vi "acquire multi waves init subvi.vi"(10 "Enum in":enum16{"Idle", "Start"}(ring), 11 "VISA Refnum in":refnum<visa-resource-name>) -> (0 "error out":errorcluster, 1 "read buffer":string, 2 "Enum out":enum16{"Idle", "Start"}(ring), 3 "VISA Refnum out":refnum<visa-resource-name>)   [LabVIEW 2013]
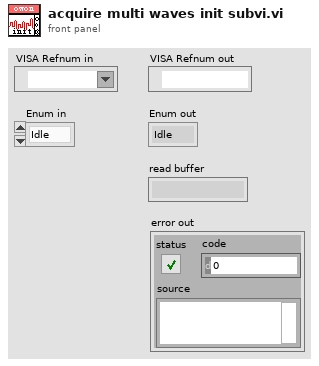
[diagram p1: front panel]
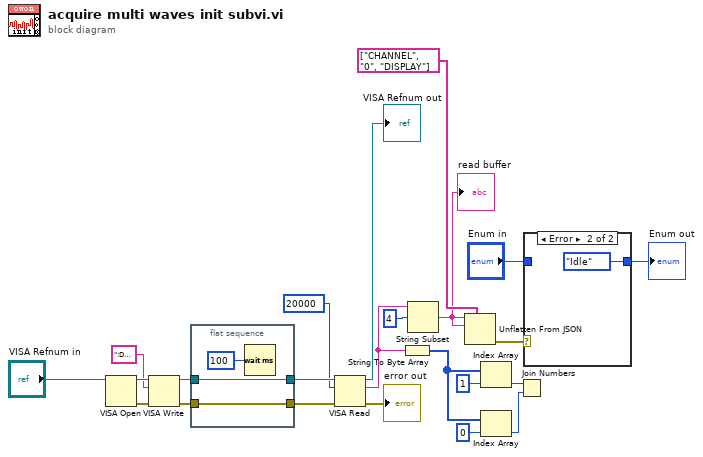
[diagram p0: block diagram]
diagram:
  n1 = VISA Open(VISA resource name="VISA Refnum in") -> (VISA resource name=w11:refnum<visa-resource-name>, error out=w12:errorcluster)  [unwired: 4 in]
  n2 = VISA Write(VISA resource name=w11, write buffer=":DATA:WAVE:SCREEN:HEAD?" ("ID Query"), error in (no error)=w12) -> (VISA resource name out=w20:refnum<visa-resource-name>, error out=w23:errorcluster)  [unwired: 1 out]
  n3 = flat-sequence {
    tunnel: w20 -> [w26]
    tunnel: [w26] -> w21
    tunnel: [w25] -> w22
    tunnel: w23 -> [w25]
    frame #0 {
      n4 = Wait (ms)(milliseconds to wait=u32 100 ("等待时间（毫秒）")) -> ()  [unwired: 1 out]
    }
  }
  n5 = VISA Read(VISA resource name=w21, byte count=u32 20000, error in (no error)=w22) -> (VISA resource name out=→"VISA Refnum out":refnum<visa-resource-name>, read buffer=w18:string, error out=→"error out":errorcluster)  [unwired: 1 out]
  n6 = String To Byte Array(string=w18) -> (unsigned byte array=w13:u8[])
  n7 = String Subset(string=w18, offset (0)=4) -> (substring=w3:string)  [unwired: 1 in]
  "read buffer" <- w3
  n8 = Unflatten From JSON(path=string[] ["CHANNEL", "0", "DISPLAY"], JSON string=w3, type and defaults=w3) -> (error out=w19:errorcluster)  [unwired: 4 in, 1 out]
  n9 = Index Array(array=w13, index=1) -> (element=w15:u8)
  n10 = Index Array(array=w13, index=0) -> (element=w14:u8)
  n11 = Join Numbers(hi=w15, lo=w14) -> ()  [unwired: 1 out]
  n12 = case shown="Error" w19 {
    tunnel: [w27 enum16{"Idle", "Start"}."Idle"] -> w9
    tunnel: "Enum in" -> [w27 _]
    frame No Error {
    }
    frame Error {
    }
  }
  "Enum out" <- w9
